vi "DigitalScope.vi"() -> ()   [LabVIEW 2018]
uses:
  <vilib>/Waveform/WDTFileIO.llb/ Write Waveform to File.vi
  <vilib>/measure/NI_MABase.lvlib
panel:
  in  "噪声CH2":enum16{"均匀白噪声", "高斯白噪声", "周期性随机噪声"}(ring) caption="噪声类型"
  in  "噪声CH1":enum16{"均匀白噪声", "高斯白噪声", "周期性随机噪声"}(ring) caption="噪声类型"
  in  "数据回放":bool
  in  "数据记录":bool
  in  "采集数据":bool
  in  "CH2signal type 2":u16(ring) caption="信号类型" items=["Sine Wave", "Triangle Wave", "Square Wave", "Sawtooth Wave"]
  in  "CH1 signal type":u16(ring) caption="信号类型" items=["Sine Wave", "Triangle Wave", "Square Wave", "Sawtooth Wave"]
  in  "时间基准 ms/div":i32(knob)=2 step=1 scale=0.0..4.0
  in  "电压基准 v/div":i32(knob)=3 step=1 scale=0.0..4.0
  in  "CH2幅度 V":dbl(knob)=2.3194908446760634 caption="幅度 V" scale=0.0..10.0
  in  "CH2频率 Hz":dbl(knob)=32.43084551092526 caption="频率 Hz" scale=0.0..200.0
  in  "CH1幅度 V":dbl(knob)=3.298875487413685 caption="幅度 V" scale=0.0..10.0
  in  "系统退出":bool
  in  "CH1频率 Hz":dbl(knob)=58.134213878999056 caption="频率 Hz" scale=0.0..200.0
  out "Waveform Graph":dynamicdata(graph)
  # "CH2"
  # "CH1"
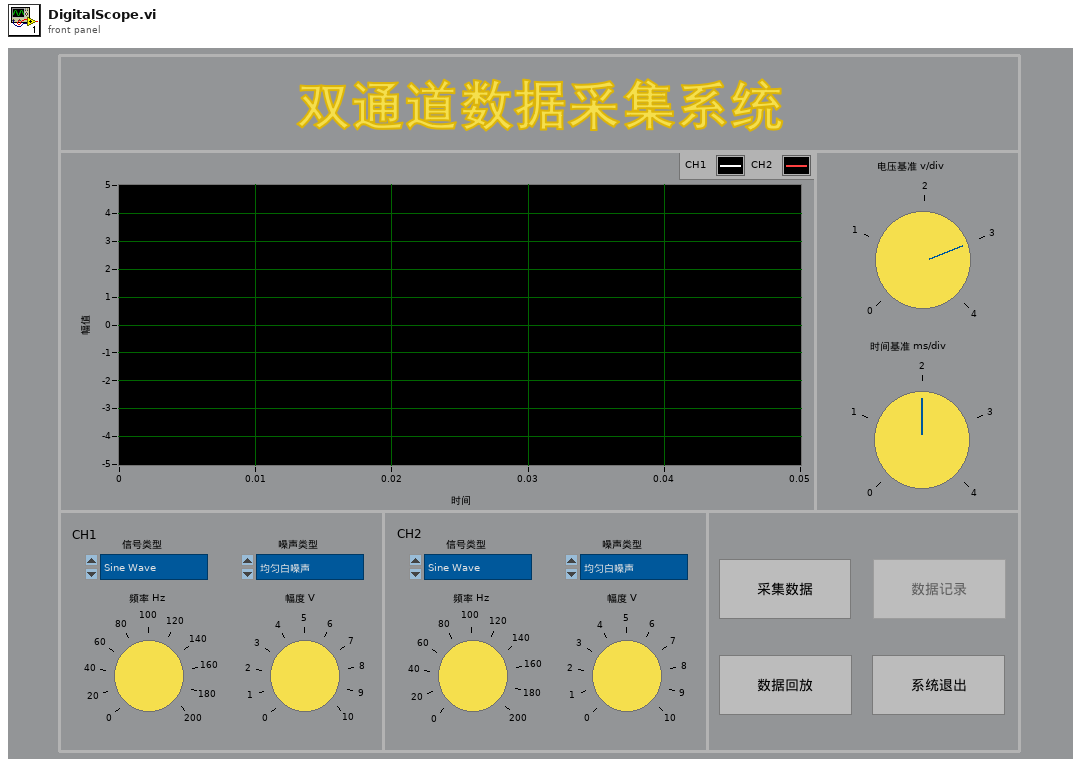
[diagram p1: front panel]
types:
  T1 = enum8{"Enabled", "Disabled", "Disabled and Grayed Out"}
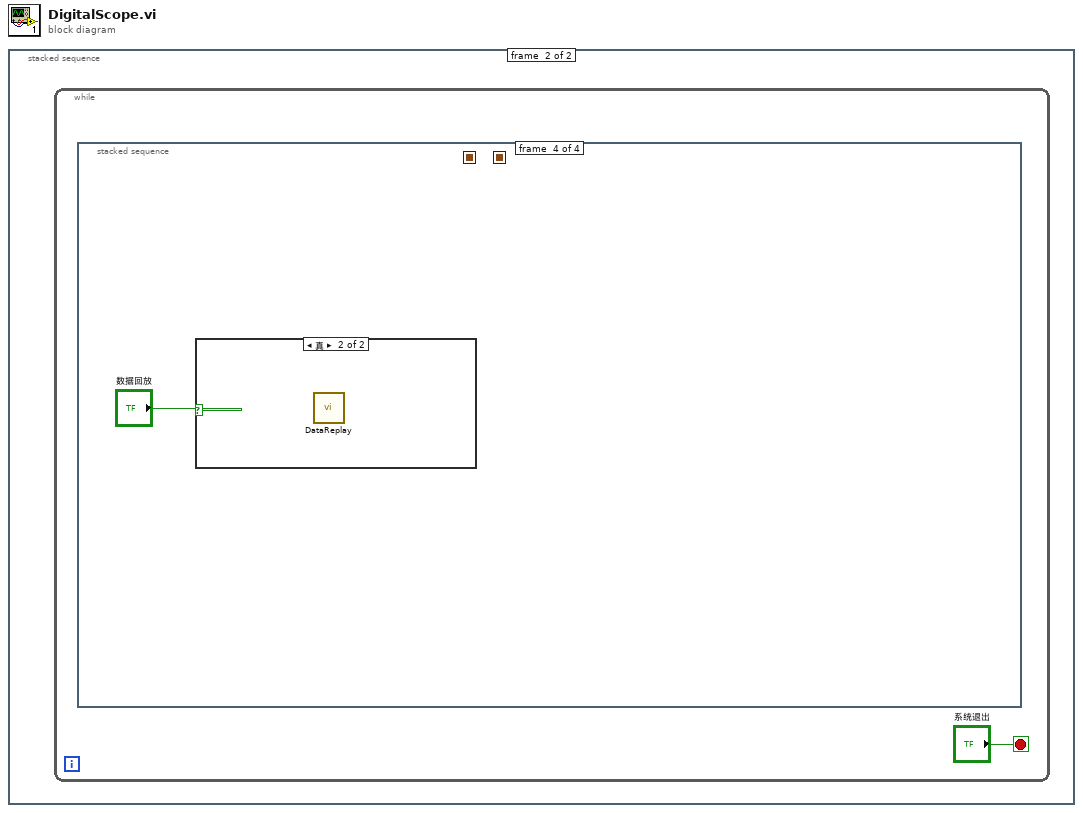
[diagram p0: block diagram]
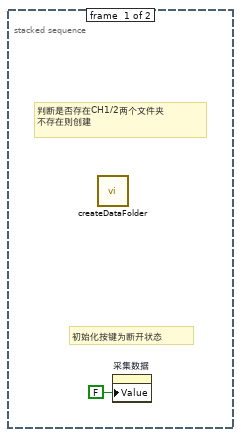
[diagram p2: hidden frame]
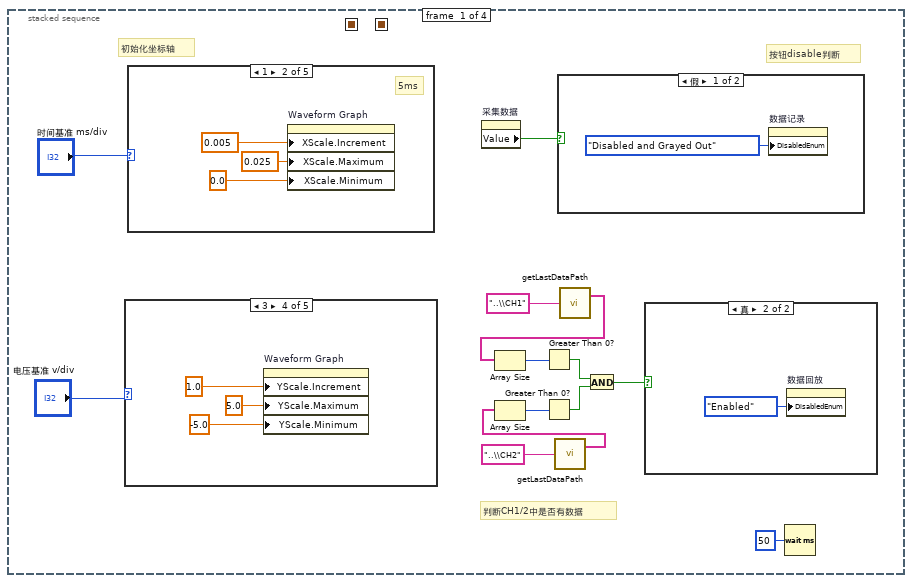
[diagram p3: hidden frame]
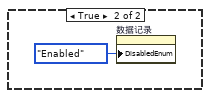
[diagram p4: hidden frame]
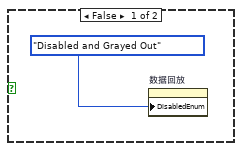
[diagram p5: hidden frame]
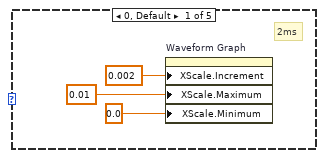
[diagram p6: hidden frame]
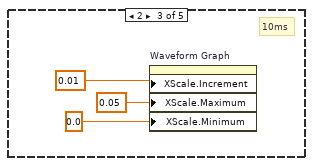
[diagram p7: hidden frame]
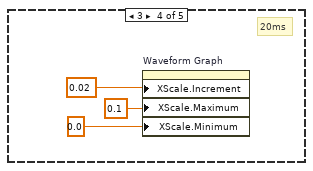
[diagram p8: hidden frame]
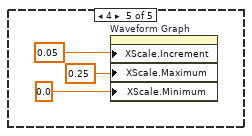
[diagram p9: hidden frame]
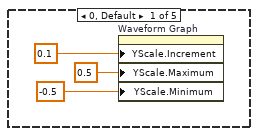
[diagram p10: hidden frame]
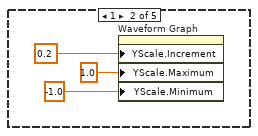
[diagram p11: hidden frame]
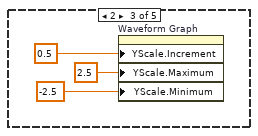
[diagram p12: hidden frame]
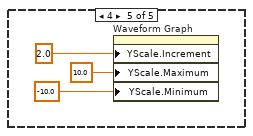
[diagram p13: hidden frame]
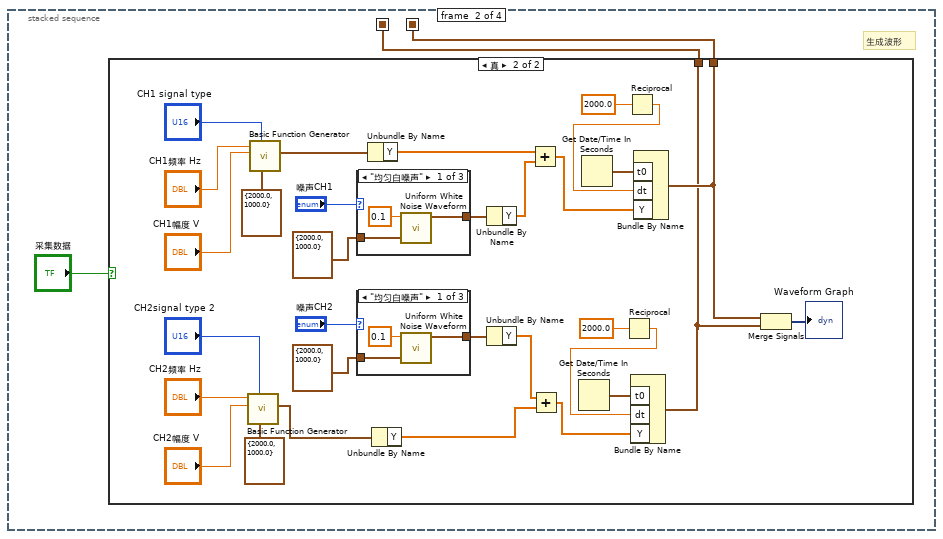
[diagram p14: hidden frame]
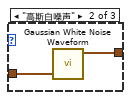
[diagram p16: hidden frame]
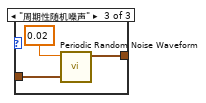
[diagram p17: hidden frame]
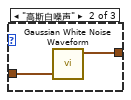
[diagram p18: hidden frame]
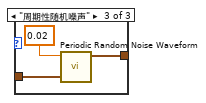
[diagram p19: hidden frame]
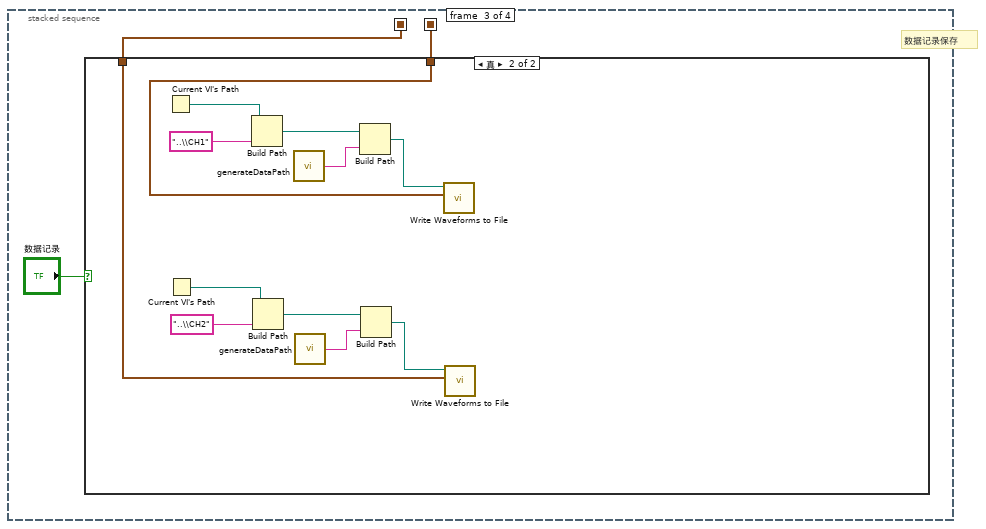
[diagram p20: hidden frame]
diagram:
  n1 = stacked-sequence {
    frame #0 {
      # "初始化按键为断开状态"
      # "判断是否存在CH1/2两个文件夹\n不存在则创建"
      n2 = call "createDataFolder.vi"() -> ()  [unwired: 12 in]
      n3 = property on="采集数据" class="Bool (严格)"("Value"=FALSE ("采集数据")) -> ()  [unwired: 2 in, 2 out]
    }
    frame #1 {
      n4 = while {
        stop <- "系统退出" stop-if-true
        n5 = stacked-sequence {
          seq-local: [_ w51 _ _] -> [_ _ w101 _]
          seq-local: [_ w50 _ _] -> [_ _ w100 _]
          frame #0 {
            # "判断CH1/2中是否有数据"
            # "按钮disable判断"
            # "初始化坐标轴"
            n6 = case shown="3" "电压基准 v/div" {
              frame 0, Default {
                n7 = property on="Waveform Graph" class="WFGraph (严格)"("YScale.Increment"=0.1 ("X标尺.范围:增量"), "YScale.Maximum"=0.5 ("X标尺.范围:最大值"), "YScale.Minimum"=-0.5 ("X标尺.范围:最小值")) -> ()  [unwired: 2 in, 2 out]
              }
              frame 1 {
                n8 = property on="Waveform Graph" class="WFGraph (严格)"("YScale.Increment"=0.2 ("X标尺.范围:增量"), "YScale.Maximum"=1.0 ("X标尺.范围:最大值"), "YScale.Minimum"=-1.0 ("X标尺.范围:最小值")) -> ()  [unwired: 2 in, 2 out]
              }
              frame 2 {
                n9 = property on="Waveform Graph" class="WFGraph (严格)"("YScale.Increment"=0.5 ("X标尺.范围:增量"), "YScale.Maximum"=2.5 ("X标尺.范围:最大值"), "YScale.Minimum"=-2.5 ("X标尺.范围:最小值")) -> ()  [unwired: 2 in, 2 out]
              }
              frame 3 {
                n10 = property on="Waveform Graph" class="WFGraph (严格)"("YScale.Increment"=1.0 ("X标尺.范围:增量"), "YScale.Maximum"=5.0 ("X标尺.范围:最大值"), "YScale.Minimum"=-5.0 ("X标尺.范围:最小值")) -> ()  [unwired: 2 in, 2 out]
              }
              frame 4 {
                n11 = property on="Waveform Graph" class="WFGraph (严格)"("YScale.Increment"=2.0 ("X标尺.范围:增量"), "YScale.Maximum"=10.0 ("X标尺.范围:最大值"), "YScale.Minimum"=-10.0 ("X标尺.范围:最小值")) -> ()  [unwired: 2 in, 2 out]
              }
            }
            n12 = case shown="1" "时间基准 ms/div" {
              frame 0, Default {
                # "2ms"
                n13 = property on="Waveform Graph" class="WFGraph (严格)"("XScale.Increment"=0.002 ("X标尺.范围:增量"), "XScale.Maximum"=0.01 ("X标尺.范围:最大值"), "XScale.Minimum"=0.0 ("X标尺.范围:最小值")) -> ()  [unwired: 2 in, 2 out]
              }
              frame 1 {
                # "5ms"
                n14 = property on="Waveform Graph" class="WFGraph (严格)"("XScale.Increment"=0.005 ("X标尺.范围:增量"), "XScale.Maximum"=0.025 ("X标尺.范围:最大值"), "XScale.Minimum"=0.0 ("X标尺.范围:最小值")) -> ()  [unwired: 2 in, 2 out]
              }
              frame 2 {
                # "10ms"
                n15 = property on="Waveform Graph" class="WFGraph (严格)"("XScale.Increment"=0.01 ("X标尺.范围:增量"), "XScale.Maximum"=0.05 ("X标尺.范围:最大值"), "XScale.Minimum"=0.0 ("X标尺.范围:最小值")) -> ()  [unwired: 2 in, 2 out]
              }
              frame 3 {
                # "20ms"
                n16 = property on="Waveform Graph" class="WFGraph (严格)"("XScale.Increment"=0.02 ("X标尺.范围:增量"), "XScale.Maximum"=0.1 ("X标尺.范围:最大值"), "XScale.Minimum"=0.0 ("X标尺.范围:最小值")) -> ()  [unwired: 2 in, 2 out]
              }
              frame 4 {
                n17 = property on="Waveform Graph" class="WFGraph (严格)"("XScale.Increment"=0.05 ("X标尺.范围:增量"), "XScale.Maximum"=0.25 ("X标尺.范围:最大值"), "XScale.Minimum"=0.0 ("X标尺.范围:最小值")) -> ()  [unwired: 2 in, 2 out]
              }
            }
            n18 = property on="采集数据" class="Bool (严格)"() -> ("Value"=w9:bool)  [unwired: 2 in, 2 out]
            n19 = call "getLastDataPath.vi"("文件夹输入"="..\\CH2") -> ("数据文件名数组"=w6:string[])  [unwired: 1 out]
            n20 = Array Size(array=w6) -> (size(s)=w7:i32)
            n21 = Greater Than 0?(x=w7) -> (x > 0?=w5:bool)
            n22 = case shown="假" w9 {
              frame False {
                n23 = property on="数据记录" class="Bool"("DisabledEnum"=T1."Disabled and Grayed Out" ("禁用")) -> ()  [unwired: 2 in, 2 out]
              }
              frame True {
                n24 = property on="数据记录" class="Bool"("DisabledEnum"=T1."Enabled" ("禁用")) -> ()  [unwired: 2 in, 2 out]
              }
            }
            n25 = call "getLastDataPath.vi"("文件夹输入"="..\\CH1") -> ("数据文件名数组"=w10:string[])  [unwired: 1 out]
            n26 = Array Size(array=w10) -> (size(s)=w11:i32)
            n27 = Greater Than 0?(x=w11) -> (x > 0?=w4:bool)
            n28 = And(x=w4, y=w5) -> (x .and. y?=w3:bool)
            n29 = case shown="真" w3 {
              frame False {
                n30 = property on="数据回放" class="Bool"("DisabledEnum"=T1."Disabled and Grayed Out" ("禁用")) -> ()  [unwired: 2 in, 2 out]
              }
              frame True {
                n31 = property on="数据回放" class="Bool"("DisabledEnum"=T1."Enabled" ("禁用")) -> ()  [unwired: 2 in, 2 out]
              }
            }
            n32 = Wait (ms)(milliseconds to wait=u32 50 ("等待时间（毫秒）")) -> ()  [unwired: 1 out]
          }
          frame #1 {
            # "生成波形"
            n33 = case shown="真" "采集数据" {
              tunnel: [_ w63] -> w51
              tunnel: [_ w59] -> w50
              frame False {
              }
              frame True {
                n34 = call <vilib>:"Basic Function Generator.vi"("sampling info"=cluster{"Fs":dbl, "#s":dbl} {"Fs"=2000.0, "#s"=1000.0}, "signal type"="CH2signal type 2", "amplitude"="CH2幅度 V", "frequency"="CH2频率 Hz") -> ("signal out"=w71:waveform(dbl))  [unwired: 5 in, 2 out]
                n35 = call <vilib>:"Basic Function Generator.vi"("sampling info"=cluster{"Fs":dbl, "#s":dbl} {"Fs"=2000.0, "#s"=1000.0}, "signal type"="CH1 signal type", "amplitude"="CH1幅度 V", "frequency"="CH1频率 Hz") -> ("signal out"=w69:waveform(dbl))  [unwired: 5 in, 2 out]
                n36 = case shown="\"均匀白噪声\"" "噪声CH1" {
                  tunnel: cluster{"Fs":dbl, "#s":dbl} {"Fs"=2000.0, "#s"=1000.0} ("sampling info") -> [w94 w95 w98]
                  tunnel: [w93 w96 w99] -> w72
                  frame "均匀白噪声" {
                    n37 = call <vilib>:"Uniform White Noise Waveform.vi"("sampling info"=w94, "amplitude"=0.1) -> ("signal out"=w93:waveform(dbl))  [unwired: 8 in, 1 out]
                  }
                  frame "高斯白噪声" {
                    n38 = call <vilib>:"Gaussian White Noise Waveform.vi"("sampling info"=w95) -> ("signal out"=w96:waveform(dbl))  [unwired: 9 in, 1 out]
                  }
                  frame "周期性随机噪声" {
                    n39 = call <vilib>:"Periodic Random Noise Waveform.vi"("sampling info"=w98, "spectral amplitude"=0.02) -> ("signal out"=w99:waveform(dbl))  [unwired: 8 in, 1 out]
                  }
                }
                n40 = case shown="\"均匀白噪声\"" "噪声CH2" {
                  tunnel: cluster{"Fs":dbl, "#s":dbl} {"Fs"=2000.0, "#s"=1000.0} ("sampling info") -> [w86 w87 w90]
                  tunnel: [w85 w88 w91] -> w55
                  frame "均匀白噪声" {
                    n41 = call <vilib>:"Uniform White Noise Waveform.vi"("sampling info"=w86, "amplitude"=0.1) -> ("signal out"=w85:waveform(dbl))  [unwired: 8 in, 1 out]
                  }
                  frame "高斯白噪声" {
                    n42 = call <vilib>:"Gaussian White Noise Waveform.vi"("sampling info"=w87) -> ("signal out"=w88:waveform(dbl))  [unwired: 9 in, 1 out]
                  }
                  frame "周期性随机噪声" {
                    n43 = call <vilib>:"Periodic Random Noise Waveform.vi"("sampling info"=w90, "spectral amplitude"=0.02) -> ("signal out"=w91:waveform(dbl))  [unwired: 8 in, 1 out]
                  }
                }
                n44 = Unbundle By Name(w69) -> ("Y"=w68:dbl[])
                n45 = Unbundle By Name(w71) -> ("Y"=w70:dbl[])
                n46 = Unbundle By Name(w72) -> ("Y"=w67:dbl[])
                n47 = Unbundle By Name(w55) -> ("Y"=w53:dbl[])
                n48 = Add(x=w68, y=w67) -> (x+y=w66:dbl[])
                n49 = Add(x=w53, y=w70) -> (x+y=w61:dbl[])
                n50 = Get Date/Time In Seconds() -> (seconds since 1Jan1904=w62:timestamp)
                n51 = Get Date/Time In Seconds() -> (seconds since 1Jan1904=w64:timestamp)
                n52 = Reciprocal(x=2000.0) -> (1/x=w60:dbl)
                n53 = Reciprocal(x=2000.0) -> (1/x=w65:dbl)
                n54 = Bundle By Name("t0"=w62, "dt"=w60, "Y"=w61) -> (w59:waveform(dbl))  [unwired: 1 in]
                n55 = Bundle By Name("t0"=w64, "dt"=w65, "Y"=w66) -> (w63:waveform(dbl))  [unwired: 1 in]
                n56 = Merge Signals(w63, w59) -> (→"Waveform Graph":dynamicdata)
              }
            }
          }
          frame #2 {
            # "数据记录保存"
            n57 = case shown="真" "数据记录" {
              tunnel: w101 -> [_ w109]
              tunnel: w100 -> [_ w103]
              frame False {
              }
              frame True {
                n58 = Current VI's Path() -> (path=w114:path)
                n59 = Current VI's Path() -> (path=w108:path)
                n60 = Build Path(base path=w114, name or relative path="..\\CH1") -> (appended path=w112:path)
                n61 = Build Path(base path=w108, name or relative path="..\\CH2") -> (appended path=w106:path)
                n62 = call "generateDataPath.vi"() -> ("连接的字符串"=w111:string)
                n63 = call "generateDataPath.vi"() -> ("连接的字符串"=w105:string)
                n64 = Build Path(base path=w112, name or relative path=w111) -> (appended path=w110:path)
                n65 = Build Path(base path=w106, name or relative path=w105) -> (appended path=w104:path)
                n66 = call-poly <vilib>:"Write Waveforms to File.vi"("waveform"=w109, "file path (dialog if empty)"=w110) -> ()  [unwired: 8 in, 2 out]
                n67 = call-poly <vilib>:"Write Waveforms to File.vi"("waveform"=w103, "file path (dialog if empty)"=w104) -> ()  [unwired: 8 in, 2 out]
              }
            }
          }
          frame #3 {
            n68 = case shown="真" "数据回放" {
              frame False {
              }
              frame True {
                n69 = call "DataReplay.vi"() -> ()  [unwired: 12 in]
              }
            }
          }
        }
      }
    }
  }
